vi "Get Config.vi"(8 "error in (no error)":errorcluster, 11 "SJ-210 in":refnum<class "SJ-210.lvclass">) -> (0 "error out":errorcluster, 1 "Config Data":variant, 3 "SJ-210 out":refnum<class "SJ-210.lvclass">)   [LabVIEW 2014, in "SJ-210.lvlib" / "SJ-210.lvclass"]
uses:
  SJ-210.lvclass
  SJ-210.lvclass/SJ-210.ctl
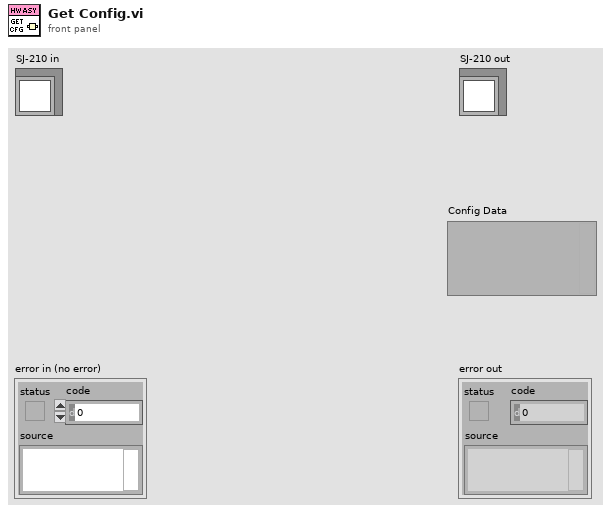
[diagram p1: front panel]
types:
  T1 = cluster{"VISA resource name":refnum<visa-resource-name>}
  T2 = cluster{"Conection Data":cluster{"VISA resource name":refnum<visa-resource-name>}, "ACQ Data":dbl[]}
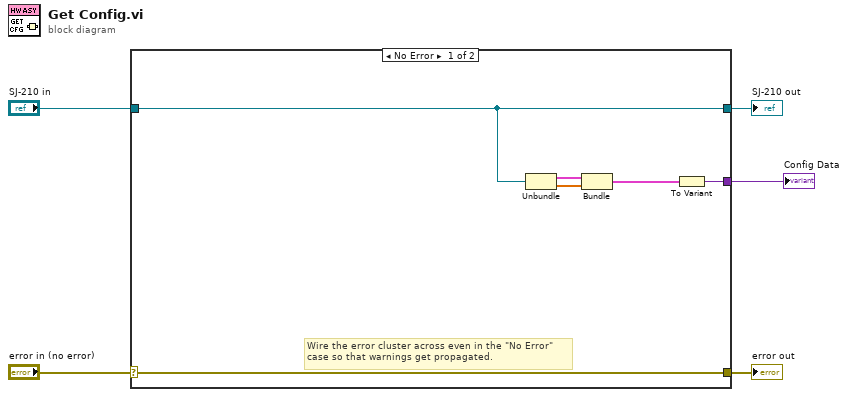
[diagram p0: block diagram]
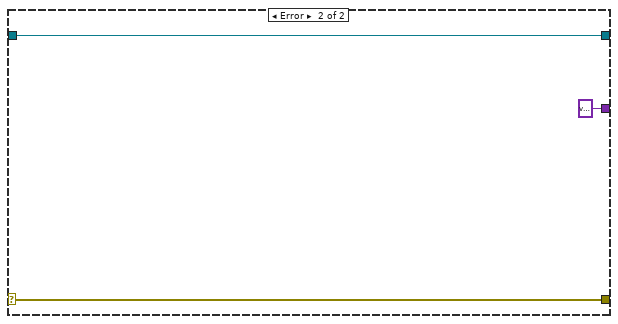
[diagram p2: hidden frame]
diagram:
  n1 = case shown="No Error" "error in (no error)" {
    selector: "error in (no error)" -> [w11 w14]
    tunnel: [w11 w14] -> w4
    tunnel: [w9 w13] -> w2
    tunnel: "SJ-210 in" -> [w9 w13]
    tunnel: [w10 variant ("Variant")] -> w1
    frame No Error {
      # "Wire the error cluster across even in the \"No Error\"\ncase so that warnings get propagated."
      n2 = Unbundle(w9) -> (w8:T1, w7:dbl[])
      n3 = Bundle("Conection Data"=w8, "ACQ Data"=w7) -> (w6:T2)  [unwired: 1 in]
      n4 = To Variant(anything=w6) -> (Variant=w10:variant)
    }
    frame Error {
    }
  }
  "error out" <- w4
  "SJ-210 out" <- w2
  "Config Data" <- w1
